vi "Post-Install Custom Action.vi"(10 "Variant":variant) -> (0 "error out":errorcluster)   [LabVIEW 2020]
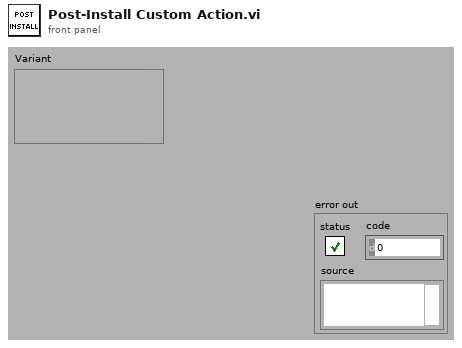
[diagram p1: front panel]
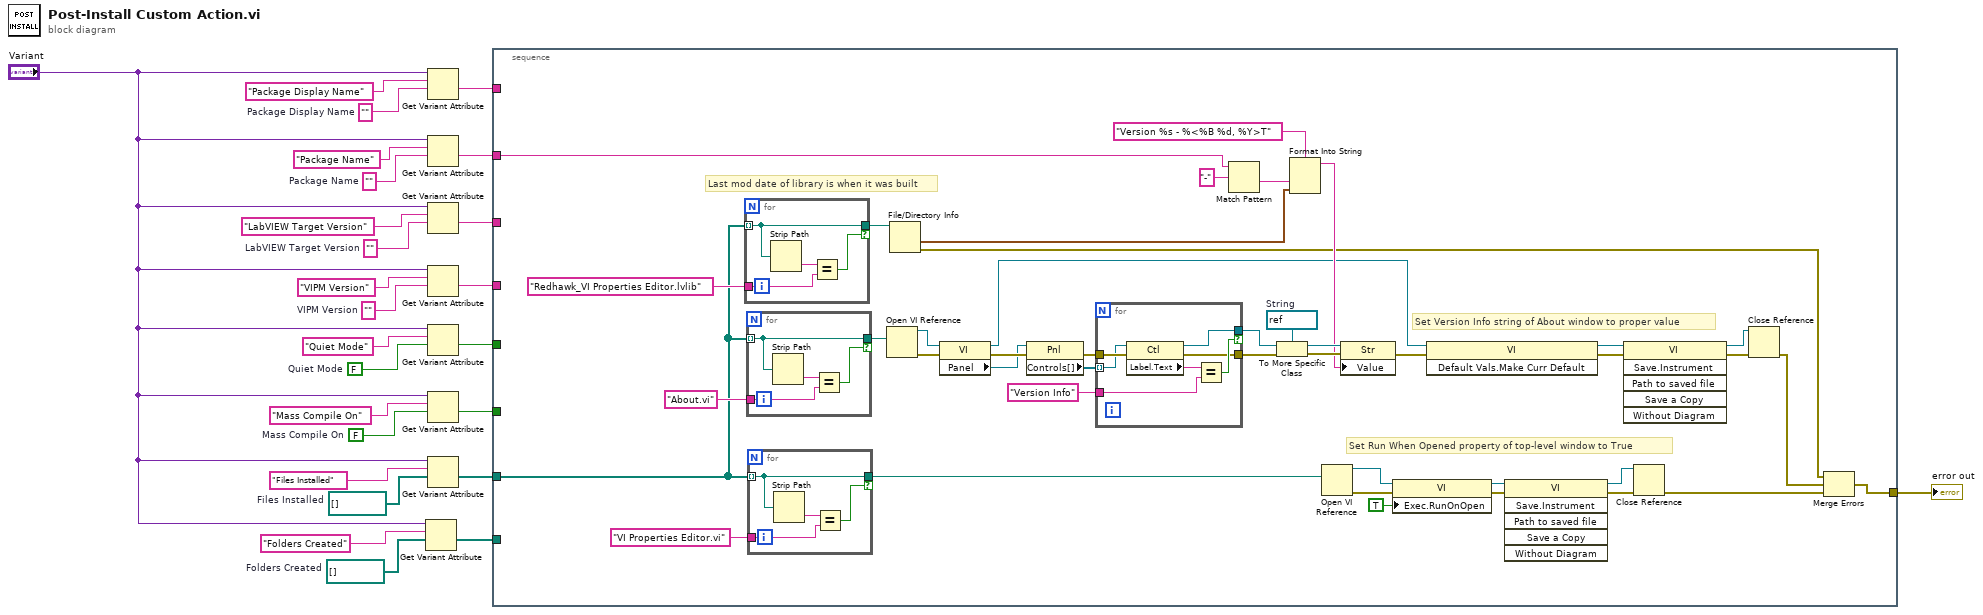
[diagram p0: block diagram]
diagram:
  w2 = path[] []  # Folders Created
  w3 = path[] []  # Files Installed
  w9 = FALSE  # Mass Compile On
  w10 = ""  # Package Display Name
  w17 = FALSE  # Quiet Mode
  w20 = ""  # VIPM Version
  w22 = ""  # LabVIEW Target Version
  w24 = ""  # Package Name
  n1 = Get Variant Attribute(Variant="Variant", name="Folders Created", default value (empty Variant)=w2) -> (value=w7:path[])  [unwired: 1 in, 3 out]
  n2 = Get Variant Attribute(Variant="Variant", name="Package Display Name", default value (empty Variant)=w10) -> (value=w16:string)  [unwired: 1 in, 3 out]
  n3 = Get Variant Attribute(Variant="Variant", name="Package Name", default value (empty Variant)=w24) -> (value=w15:string)  [unwired: 1 in, 3 out]
  n4 = Get Variant Attribute(Variant="Variant", name="LabVIEW Target Version", default value (empty Variant)=w22) -> (value=w14:string)  [unwired: 1 in, 3 out]
  n5 = Get Variant Attribute(Variant="Variant", name="VIPM Version", default value (empty Variant)=w20) -> (value=w13:string)  [unwired: 1 in, 3 out]
  n6 = Get Variant Attribute(Variant="Variant", name="Quiet Mode", default value (empty Variant)=w17) -> (value=w12:bool)  [unwired: 1 in, 3 out]
  n7 = Get Variant Attribute(Variant="Variant", name="Mass Compile On", default value (empty Variant)=w9) -> (value=w11:bool)  [unwired: 1 in, 3 out]
  n8 = Get Variant Attribute(Variant="Variant", name="Files Installed", default value (empty Variant)=w3) -> (value=w6:path[])  [unwired: 1 in, 3 out]
  n9 = stacked-sequence {
    tunnel: w16 -> [_]
    tunnel: w15 -> [w53]
    tunnel: w14 -> [_]
    tunnel: w13 -> [_]
    tunnel: w12 -> [_]
    tunnel: w11 -> [_]
    tunnel: w6 -> [w33]
    tunnel: w7 -> [_]
    tunnel: [w30] -> w1
    frame #0 {
      w40 = refnum<vi> refnum  # String
      # "Last mod date of library is when it was built"
      # "Set Version Info string of About window to proper value"
      # "Set Run When Opened property of top-level window to True"
      n10 = for {
        tunnel: w33 -> [w71] mode=indexing
        tunnel: [w71] -> w32 if=w70
        tunnel: "Redhawk_VI Properties Editor.lvlib" -> [w69]
        n11 = Strip Path(path=w71) -> (name=w72:string)  [unwired: 1 out]
        n12 = Equal?(x=w72, y=w69) -> (x = y?=w70:bool)
      }
      n13 = for {
        tunnel: w33 -> [w82] mode=indexing
        tunnel: [w82] -> w55 if=w81
        tunnel: "About.vi" -> [w80]
        n14 = Strip Path(path=w82) -> (name=w83:string)  [unwired: 1 out]
        n15 = Equal?(x=w83, y=w80) -> (x = y?=w81:bool)
      }
      n16 = for {
        tunnel: w33 -> [w86] mode=indexing
        tunnel: [w86] -> w68 if=w85
        tunnel: "VI Properties Editor.vi" -> [w84]
        n17 = Strip Path(path=w86) -> (name=w87:string)  [unwired: 1 out]
        n18 = Equal?(x=w87, y=w84) -> (x = y?=w85:bool)
      }
      n19 = Open VI Reference(vi path=w55) -> (vi reference=w48:refnum<vi>, error out=w49:errorcluster)  [unwired: 5 in]
      n20 = File/Directory Info(path=w32) -> (last mod=w31:timestamp, error out=w28:errorcluster)  [unwired: 1 in, 5 out]
      n21 = property class="VI"(reference=w48, error in=w49) -> (reference out=w36:refnum<vi>, error out=w47:errorcluster, "Panel"=w46:refnum<vi>)
      n22 = property class="Pnl"(reference=w46, error in=w47) -> (error out=w44:errorcluster, "Controls[]"=w45:refnum<vi>[])  [unwired: 1 out]
      n23 = for {
        tunnel: w45 -> [w78] mode=indexing
        tunnel: w44 -> [w79]
        tunnel: "Version Info" ("Control Name") -> [w77]
        tunnel: [w75] -> w42 if=w74
        tunnel: [w73] -> w29
        n24 = property class="Ctl"(reference=w78, error in=w79) -> (reference out=w75:refnum<vi>, error out=w73:errorcluster, "Label.Text"=w76:string)
        n25 = Equal?(x=w76, y=w77) -> (x = y?=w74:bool)
      }
      n26 = Match Pattern(string=w53, regular expression="-") -> (after substring=w50:string)  [unwired: 1 in, 3 out]
      n27 = To More Specific Class(target class=w40, reference=w42, error in=w29) -> (specific class reference=w41:refnum<vi>, error out=w39:errorcluster)
      n28 = Format Into String(format string="Version %s - %<%B %d, %Y>T", w50, w31) -> (resulting string=w37:string)  [unwired: 2 in, 1 out]
      n29 = Open VI Reference(vi path=w68) -> (vi reference=w66:refnum<vi>, error out=w67:errorcluster)  [unwired: 5 in]
      n30 = property class="Str"(reference=w41, error in=w39, "Value"=w37) -> (error out=w38:errorcluster)  [unwired: 1 out]
      n31 = property class="VI"(reference=w66, error in=w67, "Exec.RunOnOpen"=TRUE ("Execution:Run When Opened")) -> (reference out=w63:refnum<vi>, error out=w64:errorcluster)
      n32 = invoke class="VI" method="Default Vals.Make Curr Default"(reference=w36, error in=w38) -> (reference out=w35:refnum<vi>, error out=w54:errorcluster)  [unwired: 1 in, 1 out]
      n33 = invoke class="VI" method="Save.Instrument"(reference=w63, error in=w64) -> (reference out=w61:refnum<vi>, error out=w62:errorcluster)  [unwired: 4 in, 4 out]
      n34 = invoke class="VI" method="Save.Instrument"(reference=w35, error in=w54) -> (reference out=w57:refnum<vi>, error out=w56:errorcluster)  [unwired: 4 in, 4 out]
      n35 = Close Reference(reference=w61, error in (no error)=w62) -> (error out=w60:errorcluster)
      n36 = Close Reference(reference=w57, error in (no error)=w56) -> (error out=w27:errorcluster)
      n37 = Merge Errors(w28, w27, w60) -> (w30:errorcluster)
    }
  }
  "error out" <- w1
